vi ".NET Type Builder Struct Layout Attribute.vi"(8 "error in (no error)":errorcluster, 9 "Char Set":i32(ring)=4 items=["None"=1, "Ansi"=2, "Unicode"=3, "Auto"=4], 10 "Pack Size":i32(ring)=8 items=["Unspecified"=0, "Size1"=1, "Size2"=2, "Size4"=4, "Size8"=8, "Size16"=16, "Size32"=32, "Size64"=64, "Size128"=128], 11 "Layout Kind":i32(ring) items=["Sequential"=0, "Explicit"=2, "Auto"=3]) -> (0 "error out":errorcluster, 1 ".NET Custom Attribute Builder":refnum<k24>)   [LabVIEW 2018, in "TwinCAT ADS.lvclass"]
uses:
  TwinCAT ADS.lvclass
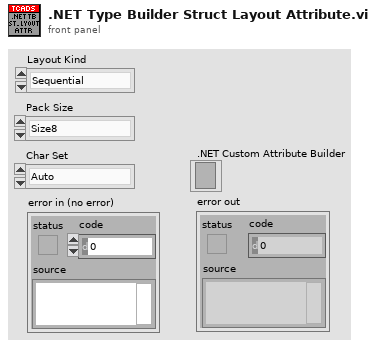
[diagram p1: front panel]
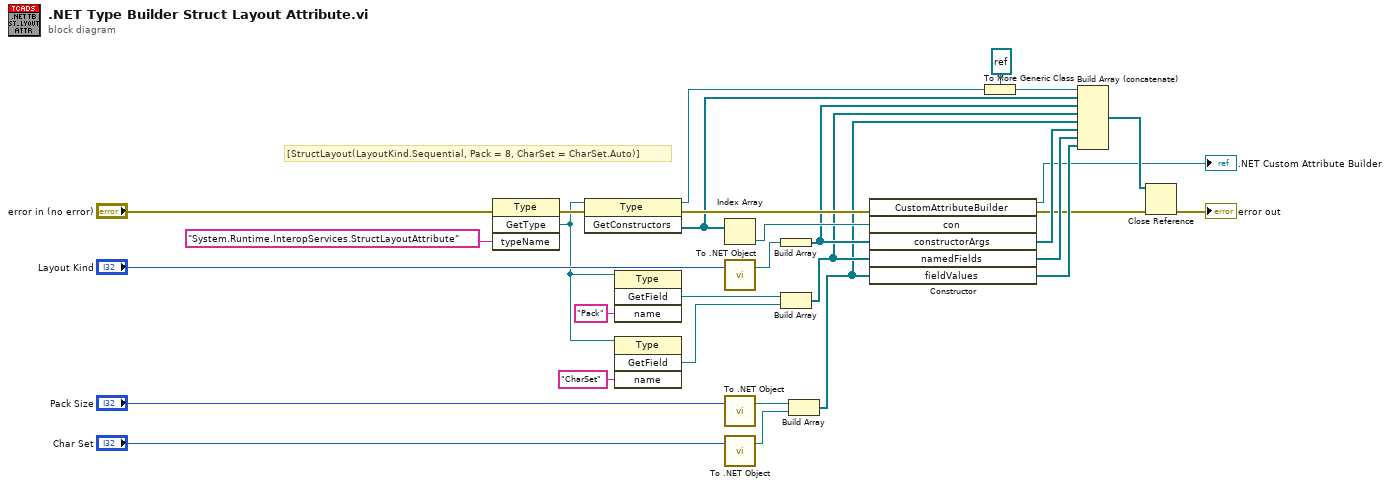
[diagram p0: block diagram]
diagram:
  # "[StructLayout(LayoutKind.Sequential, Pack = 8, CharSet = CharSet.Auto)]"
  n1 = invoke class="Type" method="GetType"(error in="error in (no error)", "typeName"="System.Runtime.InteropServices.StructLayoutAttribute" ("assemblyName")) -> (error out=w29:errorcluster, "GetType"=w22:refnum<k24>)  [unwired: 2 in, 2 out]
  n2 = invoke class="Type" method="GetConstructors"(reference=w22, error in=w29) -> (reference out=w12:refnum<k24>, error out=w27:errorcluster, "GetConstructors"=w9:refnum<k24>[])  [unwired: 1 in]
  n3 = invoke class="Type" method="GetField"(reference=w22, "name"="Pack") -> ("GetField"=w21:refnum<k24>)  [unwired: 2 in, 3 out]
  n4 = invoke class="Type" method="GetField"(reference=w22, "name"="CharSet") -> ("GetField"=w20:refnum<k24>)  [unwired: 2 in, 3 out]
  n5 = Index Array(array=w9) -> (element=w28:refnum<k24>)  [unwired: 1 in]
  n6 = call <vilib>:"To .NET Object.vi"("anything"="Layout Kind") -> (".NET object"=w25:refnum<k24>)  [unwired: 1 in, 1 out]
  n7 = call <vilib>:"To .NET Object.vi"("anything"="Pack Size") -> (".NET object"=w19:refnum<k24>)  [unwired: 1 in, 1 out]
  n8 = call <vilib>:"To .NET Object.vi"("anything"="Char Set") -> (".NET object"=w17:refnum<k24>)  [unwired: 1 in, 1 out]
  n9 = Build Array(w25) -> (w8:refnum<k24>[])
  n10 = Build Array(w21, w20) -> (w7:refnum<k24>[])
  n11 = Build Array(w19, w17) -> (w6:refnum<k24>[])
  n12 = constructor class="CustomAttributeBuilder"(error in=w27, "con"=w28, "constructorArgs"=w8, "namedFields"=w7, "fieldValues"=w6) -> (reference out=→".NET Custom Attribute Builder":refnum<k24>, error out=w5:errorcluster, "constructorArgs"=w15:refnum<k24>[], "namedFields"=w14:refnum<k24>[], "fieldValues"=w13:refnum<k24>[])  [unwired: 2 in, 2 out]
  n13 = To More Generic Class(target class=refnum<k24> refnum ("DefineType"), reference=w12) -> (generic class reference=w10:refnum<k24>)
  n14 = Build Array (concatenate)(w10, w9, w8, w7, w6, w15, w14, w13) -> (w4:refnum<k24>[])
  n15 = Close Reference(reference=w4, error in (no error)=w5) -> (error out=→"error out":errorcluster)
